vi "Average or Samples check results.vi"(4 "Array":dbl[](array[numeric]), 6 "Average(True)\nor Samples(False)":bool, 8 "In Range (True)\nor Max (False)":bool, 9 "Accurrance.\n(unused for Max check)":dbl, 10 "Dec (True) or\nHex (False)":bool, 11 "Value (or Max value)":dbl) -> (1 "String":string, 3 "Results OK ?":bool)   [LabVIEW 2017]
panel:
  in  "Always show\naverage":bool=TRUE
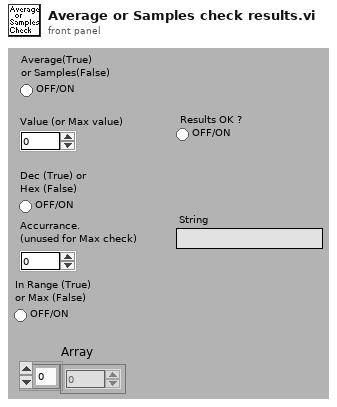
[diagram p1: front panel]
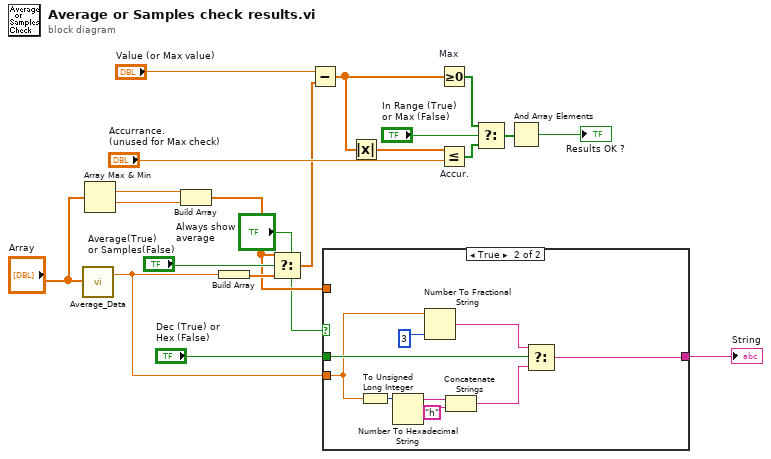
[diagram p0: block diagram]
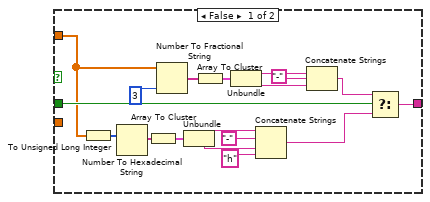
[diagram p2: hidden frame]
diagram:
  n1 = call "Average_Data.vi"("Data in"="Array") -> ("Average DBL"=w3:dbl)  [unwired: 1 out]
  n2 = Array Max & Min(array="Array") -> (max value=w10:dbl, min value=w9:dbl)  [unwired: 2 out]
  n3 = Build Array(w10, w9) -> (w2:dbl[])
  n4 = Build Array(w3) -> (w8:dbl[])
  n5 = Select(t=w2, s="Average(True)\nor Samples(False)", f=w8) -> (s? t:f=w7:dbl[])
  n6 = Subtract(x="Value (or Max value)", y=w7) -> (x-y=w13:dbl[])
  n7 = case shown="True" "Always show\naverage" {
    tunnel: [w38 w47] -> w20
    tunnel: "Dec (True) or\nHex (False)" -> [w35 w46]
    tunnel: w3 -> [_ w39]
    tunnel: w2 -> [w32 _]
    frame False {
      n8 = To Unsigned Long Integer(number=w32) -> (unsigned 32bit integer=w37:u32[])
      n9 = Number To Hexadecimal String(2:w37) -> (0:w34:string[])  [unwired: 1 in]
      n10 = Array To Cluster(array=w34) -> (cluster=w33:cluster{"[0]":string, "[1]":string})
      n11 = Number To Fractional String(number=w32, precision (6)=i16 3) -> (F-format string=w26:string[])  [unwired: 2 in]
      n12 = Unbundle(w33) -> ("[0]"=w31:string, "[1]"=w29:string)
      n13 = Array To Cluster(array=w26) -> (cluster=w27:cluster{"[0]":string, "[1]":string})
      n14 = Unbundle(w27) -> ("[0]"=w24:string, "[1]"=w23:string)
      n15 = Concatenate Strings(w31, "-", w29, "h") -> (w21:string)
      n16 = Concatenate Strings(w24, "-", w23) -> (w22:string)
      n17 = Select(t=w22, s=w35, f=w21) -> (s? t:f=w38:string)
    }
    frame True {
      n18 = To Unsigned Long Integer(number=w39) -> (unsigned 32bit integer=w41:u32)
      n19 = Number To Hexadecimal String(2:w41) -> (0:w42:string)  [unwired: 1 in]
      n20 = Number To Fractional String(number=w39, precision (6)=i16 3) -> (F-format string=w45:string)  [unwired: 2 in]
      n21 = Concatenate Strings(w42, "h" ("string")) -> (w44:string)
      n22 = Select(t=w45, s=w46, f=w44) -> (s? t:f=w47:string)
    }
  }
  "String" <- w20
  n23 = Absolute Value(x=w13) -> (abs(x)=w12:dbl[])
  n24 = Greater Or Equal To 0? "Max"(x=w13) -> (x >= 0?=w14:bool[])
  n25 = Less Or Equal? "Accur."(x=w12, y="Accurrance.\n(unused for Max check)") -> (x <= y?=w19:bool[])
  n26 = Select(t=w14, s="In Range (True)\nor Max (False)", f=w19) -> (s? t:f=w18:bool[])
  n27 = And Array Elements(Boolean array=w18) -> (logical AND=→"Results OK ?":bool)
